vi "Periodic Tasks.vi"(8 "error in":errorcluster) -> ()   [LabVIEW 2012]
doc: "This VI runs in parallel to other tasks. It can contain as many user-defined periodic loops as you need. These can carry out PID or other sorts of timed response."
uses:
  <vilib>/Rock Robotics/WPI/DriverStation/DriverStationLCD/WPI_DriverStationLCDLCDLine.ctl
  <vilib>/Rock Robotics/SystemInterfaces/Utilities/FPGA_UtilitiesLED Source.ctl
  <vilib>/Rock Robotics/SystemInterfaces/Utilities/FPGA_UtilitiesLED State.ctl
  Robot Global Data.vi
  <vilib>/Rock Robotics/WPI/RobotDrive/WPI_RobotDriveGetSetRefNum.vi
  <vilib>/Rock Robotics/WPI/Joystick/WPI_JoystickGetSetRefNum.vi
  <vilib>/Rock Robotics/WPI/Solenoid/Deprecated/WPI_SolenoidSetBool.vi
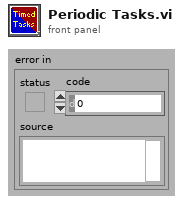
[diagram p1: front panel]
types:
  T1 = typedef "FPGA_UtilitiesLED State.ctl" = enum16{"Off", "On", "Toggle"}
  T2 = typedef "FPGA_UtilitiesLED Source.ctl" = enum16{"User LED", "FPGA LED"}
  T3 = typedef "WPI_JoystickDevRef.ctl" = cluster{"Device":T4}
  T4 = typedef "WPI_JoystickDeviceEnum.ctl" = enum16{"USB 1", "USB 2", "USB 3", "USB 4", "Kinect 1", "Kinect 2"}
  T5 = typedef "WPI_RobotDriveDevRef.ctl" = cluster{"DevStatus":errorcluster, "Motors[]":T6[], "Square Inputs":bool, "Max Output":dbl, "Isochronous":bool}
  T6 = typedef "WPI_MotorControlDeviceRef.ctl" = cluster{"DeviceStatus":errorcluster, "Type":enum16{"PWM", "CAN"}, "PWM":cluster{"Digital Module":T7, "PWM Channel":T8, "DeadBand":T9}, "CAN":cluster{"Device Number":u8, "Control Mode":T10, "Semaphore":T11, "Max Vout":dbl}, "Invert":bool, "TransformRef":T12, "InvTransformRef":T12}
  T7 = typedef "FPGA_TypedefDigitalModule.ctl" = enum16{"Digital Module 1", "Digital Module 2"}
  T8 = typedef "FPGA_DIOPWMChannel.ctl" = enum8{"PWM 1", "PWM 2", "PWM 3", "PWM 4", "PWM 5", "PWM 6", "PWM 7", "PWM 8", "PWM 9", "PWM 10", "Invalid"}
  T9 = typedef "WPI_PWMDeadband.ctl" = cluster{"Name":string, "maxPositivePwm":i32, "minPositivePwm":i32, "centerPwm":i32, "maxNegativePwm":i32, "minNegativePwm":i32, "angularRange":u16}
  T10 = typedef "WPI_CANJaguar_ControlMode.ctl" = enum8{"Percent VBus", "Current", "Speed", "Position", "Voltage"}
  T11 = typedef "Semaphore RefNum" = refnum<k1>
  T12 = typedef "WPI_PWMTransform_ConPane.ctl" = refnum<vi>
  T13 = typedef "WPI_EncoderDevRef.ctl" = cluster{"DevStatus":errorcluster, "EncoderIndex":T14, "CounterIndex":T15, "DistancePerCount":dbl, "Decoding Type":T16}
  T14 = typedef "FPGA_EncoderIdx.ctl" = enum8{"Enc 0", "Enc 1", "Enc 2", "Enc 3", "Invalid"}
  T15 = typedef "FPGA_CounterCtrSystemIndex.ctl" = enum8{"Ctr 0", "Ctr 1", "Ctr 2", "Ctr 3", "Ctr 4", "Ctr 5", "Ctr 6", "Ctr 7", "Invalid"}
  T16 = typedef "WPI_EncoderType.ctl" = enum16{"1x", "2x", "4x"}
  T17 = cluster{"JoystickDevRef":T3, "RobotDriveDevRef":T5}
  T18 = typedef "WPI_SolenoidDevRef.ctl" = cluster{"DevStatus":errorcluster, "Solenoid Module":T19, "Forward Solenoid Channel":T20, "Reverse Solenoid Channel":T20}
  T19 = typedef "FPGA_TypedefSolenoidModule.ctl" = enum16{"Solenoid Module 1", "Solenoid Module 2"}
  T20 = typedef "WPI_SolenoidChannel.ctl" = enum8{"Solenoid 1", "Solenoid 2", "Solenoid 3", "Solenoid 4", "Solenoid 5", "Solenoid 6", "Solenoid 7", "Solenoid 8", "Invalid"}
  T21 = typedef "WPI_DriverStationLCDLCDLine.ctl" = enum16{"Main - Line 1", "User - Line 2", "User - Line 3", "User - Line 4", "User - Line 5", "User - Line 6"}
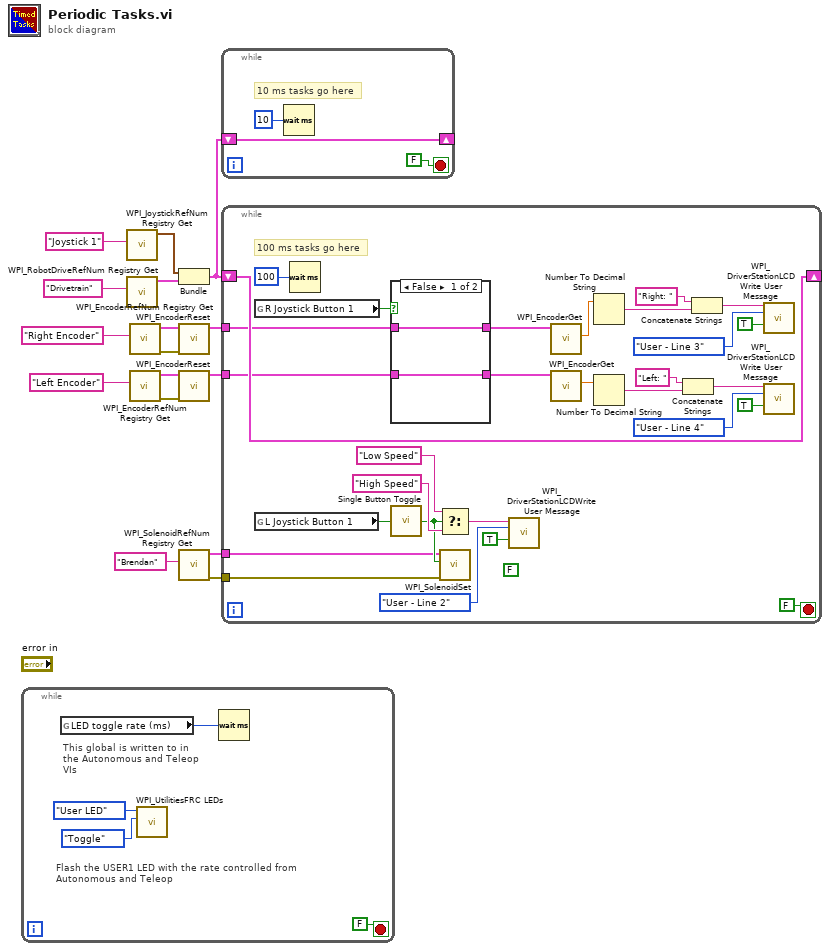
[diagram p0: block diagram]
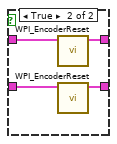
[diagram p2: hidden frame]
diagram:
  n1 = while {
    stop <- FALSE stop-if-true
    # "This global is written to in the Autonomous and Teleop VIs"
    # "Flash the USER1 LED with the rate controlled from Autonomous and Teleop"
    n2 = global read "Robot Global Data.vi" "LED toggle rate (ms)"() -> (w17:u32)
    n3 = call <vilib>:"WPI_UtilitiesFRC LEDs.vi"("State"=FPGA_UtilitiesLED_State."Toggle", "LED Type"=FPGA_UtilitiesLED_Source."User LED") -> ()  [unwired: 1 in, 9 out]
    n4 = Wait (ms)(milliseconds to wait=w17) -> ()  [unwired: 1 out]
  }
  n5 = call <vilib>:"WPI_JoystickRefNum Registry Get.vi"("refnum name"="Joystick 1") -> ("JoystickDevRef"=w14:T3)  [unwired: 1 in, 9 out]
  n6 = call <vilib>:"WPI_RobotDriveRefNum Registry Get.vi"("refnum name"="Drivetrain") -> ("RobotDriveDevRef"=w13:T5)  [unwired: 1 in, 9 out]
  n7 = call <vilib>:"WPI_EncoderRefNum Registry Get.vi"("refnum name"="Right Encoder") -> ("error out"=w11:errorcluster, "EncoderDevRef"=w10:T13)  [unwired: 9 in]
  n8 = call <vilib>:"WPI_EncoderRefNum Registry Get.vi"("refnum name"="Left Encoder") -> ("error out"=w9:errorcluster, "EncoderDevRef"=w8:T13)  [unwired: 9 in]
  n9 = Bundle("JoystickDevRef"=w14, "RobotDriveDevRef"=w13) -> (w12:T17)  [unwired: 1 out]
  n10 = call <vilib>:"WPI_EncoderReset.vi"("error in (no error)"=w11, "EncoderDevRef"=w10) -> ("EncoderDevRef"=w4:T13)  [unwired: 8 in, 1 out]
  n11 = call <vilib>:"WPI_EncoderReset.vi"("error in (no error)"=w9, "EncoderDevRef"=w8) -> ("EncoderDevRef"=w5:T13)  [unwired: 8 in, 1 out]
  n12 = call <vilib>:"WPI_SolenoidRefNum Registry Get.vi"("refnum name"="Brendan") -> ("error out"=w1:errorcluster, "SolenoidDevRef"=w2:T18)  [unwired: 9 in]
  n13 = while {
    shift-right: [w21] -> _
    shift-left: w12 -> [w21]
    stop <- FALSE stop-if-true
    # "10 ms tasks go here"
    n14 = Wait (ms)(milliseconds to wait=u32 10) -> ()  [unwired: 1 out]
  }
  n15 = while {
    shift-right: [w50] -> _
    shift-left: w12 -> [w50]
    tunnel: w5 -> [w34]
    tunnel: w4 -> [w33]
    tunnel: w2 -> [w25]
    tunnel: w1 -> [w24]
    stop <- FALSE stop-if-true
    (unwired) FALSE
    # "100 ms tasks go here"
    n16 = global read "Robot Global Data.vi" "R Joystick Button 1"() -> (w35:bool)
    n17 = global read "Robot Global Data.vi" "L Joystick Button 1"() -> (w32:bool)
    n18 = Wait (ms)(milliseconds to wait=u32 100) -> ()  [unwired: 1 out]
    n19 = case shown="False" w35 {
      tunnel: w33 -> [w53 w58]
      tunnel: [w53 w57] -> w37
      tunnel: [w54 w56] -> w36
      tunnel: w34 -> [w54 w55]
      frame False {
      }
      frame True {
        n20 = call <vilib>:"WPI_EncoderReset.vi"("EncoderDevRef"=w58) -> ("EncoderDevRef"=w57:T13)  [unwired: 9 in, 1 out]
        n21 = call <vilib>:"WPI_EncoderReset.vi"("EncoderDevRef"=w55) -> ("EncoderDevRef"=w56:T13)  [unwired: 9 in, 1 out]
      }
    }
    n22 = call "Single Button Toggle.vi"("Shoot Button 3"=w32) -> ("Boolean"=w26:bool)
    n23 = Select(t="Low Speed" ("line text"), s=w26, f="High Speed" ("line text")) -> (s? t:f=w27:string)
    n24 = call-poly <vilib>:"WPI_SolenoidSet.vi"("error in (no error)"=w24, "Value"=w26, "SolenoidDevRef"=w25) -> ()  [unwired: 7 in, 2 out]
    n25 = call <vilib>:"WPI_DriverStationLCDWrite User Message.vi"("line text"=w27, "line"=WPI_DriverStationLCDLCDLine."User - Line 2", "clear line before write (T)"=TRUE) -> ()  [unwired: 12 in, 1 out]
    n26 = call <vilib>:"WPI_EncoderGet.vi"("EncoderDevRef"=w37) -> ("Distance"=w47:dbl)  [unwired: 5 in, 5 out]
    n27 = call <vilib>:"WPI_EncoderGet.vi"("EncoderDevRef"=w36) -> ("Distance"=w38:dbl)  [unwired: 5 in, 5 out]
    n28 = Number To Decimal String(number=w47) -> (decimal integer string=w46:string)  [unwired: 1 in]
    n29 = Number To Decimal String(number=w38) -> (decimal integer string=w41:string)  [unwired: 1 in]
    n30 = Concatenate Strings("Left: ", w41) -> (w40:string)
    n31 = Concatenate Strings("Right: ", w46) -> (w44:string)
    n32 = call <vilib>:"WPI_DriverStationLCDWrite User Message.vi"("line text"=w44, "line"=WPI_DriverStationLCDLCDLine."User - Line 3", "clear line before write (T)"=TRUE) -> ()  [unwired: 12 in, 1 out]
    n33 = call <vilib>:"WPI_DriverStationLCDWrite User Message.vi"("line text"=w40, "line"=WPI_DriverStationLCDLCDLine."User - Line 4", "clear line before write (T)"=TRUE) -> ()  [unwired: 12 in, 1 out]
  }
